vi "Maximum Corr coeff.vi"() -> (5 "Plug in titles":string[](array[string]), 7 "Plug in values":string[](array[string]))   [LabVIEW 2021]
uses:
  Controls/Inst_type.ctl
  <vilib>/Analysis/3filter.llb/Filter Passband Type.ctl
  Globals/Meas_global.vi
  <vilib>/Analysis/3filter.llb/Zero Phase Filter (Cascade, DBL).vi
  <vilib>/Analysis/NI_AALBase.lvlib
panel:
  in  "Inst 2":bool
  in  "X Displacement (mm)":dbl
  out "Values":string[](array[string])
  out "Ch Names":string[](array[string])
  in  "Device ID Contains":string="B2"
  in  "Inject Sync Delay Values":bool
  in  "Minimum Correlation Coefficient\nto give time lag for":dbl=0.1
  in  "Time Trace":bool
  in  "Wind turbine location\n(Applicable only if \nInput own variables? is OFF)":dbl=10000.0
  out "Error":i32
  in  "Filter 2nd Instrument data?":bool
  in  "Freq Cutoff Inst 2":dbl=100.0
  in  "Freq Cutoff Inst 1":dbl=100.0
  in  "Filter 1st Instrument Data?":bool
  in  "Start point(s)":dbl=-1.5
  in  "Time step (s)":dbl=0.05
  in  "Input own variables?":bool=TRUE
  out "Start point":dbl
  out "XY Graph 2":cluster{dbl[], dbl[]}(graph)
  out "Time step":dbl
  in  "Number of estimates":i32=60
  out "Time Trace":cluster{"Time (ms)":dbl[], "Eng Values":dbl[]}[](graph)
  in  "Instrumnt 2":i32=1
  in  "Instrument 1":i32
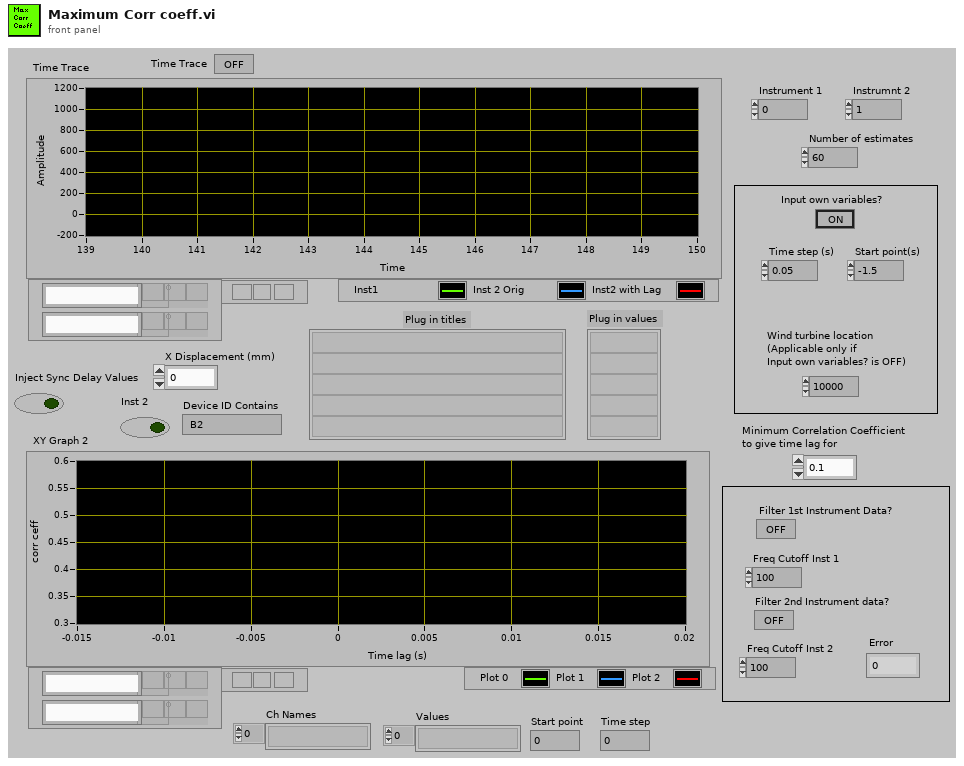
[diagram p1: front panel]
types:
  T1 = typedef "Analysis_info_cluster.ctl" = cluster{"Colour":u32, "Inst type":T2, "Inst name":string, "Symbol":string, "Code name":string, "Extra Info":string, "Inst Array":T3, "Extra Titles":string[], "Extra Values":string[], "U":dbl, "u^2":dbl, "u^3":dbl, "u^4":dbl, "Skew_u":dbl, "Kurt_u":dbl, "Sd Error in Mean":dbl, "% u'/U":dbl, "X":dbl, "Y":dbl, "Z":dbl, "Timescale integral Estimate":dbl, "Sd Error in Variance":dbl, "Calib File":path, "Calib Constants":dbl[], "Output Position":bool, "Stats":enum16{"None", "Basic", "Full"}, "Av Sampling Rate":dbl, "Av No of Samples":dbl, "Total Meas Time (s)":dbl, "ADAM Ch Name":string, "Max value":dbl, "Min value":dbl, "Req Sample Rate Hz":dbl, "Sync Delay Time (s)":dbl, "Ch No":i16, "Device":string, "Use Latest Calib":bool, "Port":string, "Metadata Ch Names":string[], "Metadata Ch Values":string[], "Label":string}
  T2 = typedef "Inst_type.ctl" = enum16{"Raw voltage", "Raw with zero offsetting", "Propeller anemometer", "Pressure Transducer", "Pitot-static tube", "Hot wire", "Cross wire 1", "Cross wire 2", "Generic Linear", "Generic Polynomial", "Generic BackPoly", "Fast FID", "Thermocouple", "Cold wire", "Pulsed Wire", "LDA Vel", "LDA Tran time", "LDA Arr time", "Microphone"}
  T3 = typedef "Instrument_Array.ctl" = enum16{"PWA", "LDA", "Analogue"}
  T4 = typedef "Time_Trace_Cluster.ctl" = cluster{"Weighting":dbl[], "Voltage":dbl[], "Eng Values":dbl[]}
  T5 = enum16{"Save no data", "Save data in new files", "Save data in existing files"}
  T6 = typedef "NI_AALBase.lvlib/Filter Passband Type.ctl" = enum32{"Lowpass", "Highpass", "Bandpass", "Bandstop"}
  T7 = cluster{"sorted array":dbl[], "Eng Values":dbl[]}
  T8 = cluster{"filter structure":enum32{"IIR 2nd Order", "IIR 4th Order"}, "Reverse Coefficients":dbl[], "Forward Coefficients":dbl[]}
  T9 = typedef "Cross_Moments_Shift_Cluster.ctl" = cluster{"Stats":dbl[], "Resampled No of Samples":i32, "Resampled delta T":dbl, "Cross Correlation":dbl[]}
  T10 = typedef "Shift_Cluster.ctl" = cluster{"Stats":dbl[], "Spectra_Auto":dbl[], "Histogram":dbl[], "Hist Max":dbl, "Hist Min":dbl, "No of Samples":i32, "No in plume":i32, "Weight sum":dbl, "No Of Hist bins":i32, "TimeTrace Max":dbl, "Time Trace Min":dbl, "Trace St Deviation":dbl}
  T11 = typedef "Correlation_cluster1.ctl" = cluster{"U inst":string, "uw":dbl, "u^2w":dbl, "uw^2":dbl, "uw/u'w'":dbl, "W inst":string, "uw^3":dbl, "u^3w":dbl, "u^2w^2":dbl, "Index U":i32, "Index W":i32, "Error info":string[], "Paired Sampling Rate (Hz)":dbl, "u^2 Paired":dbl, "w^2 Paired":dbl, "Time Window (ms)":dbl}
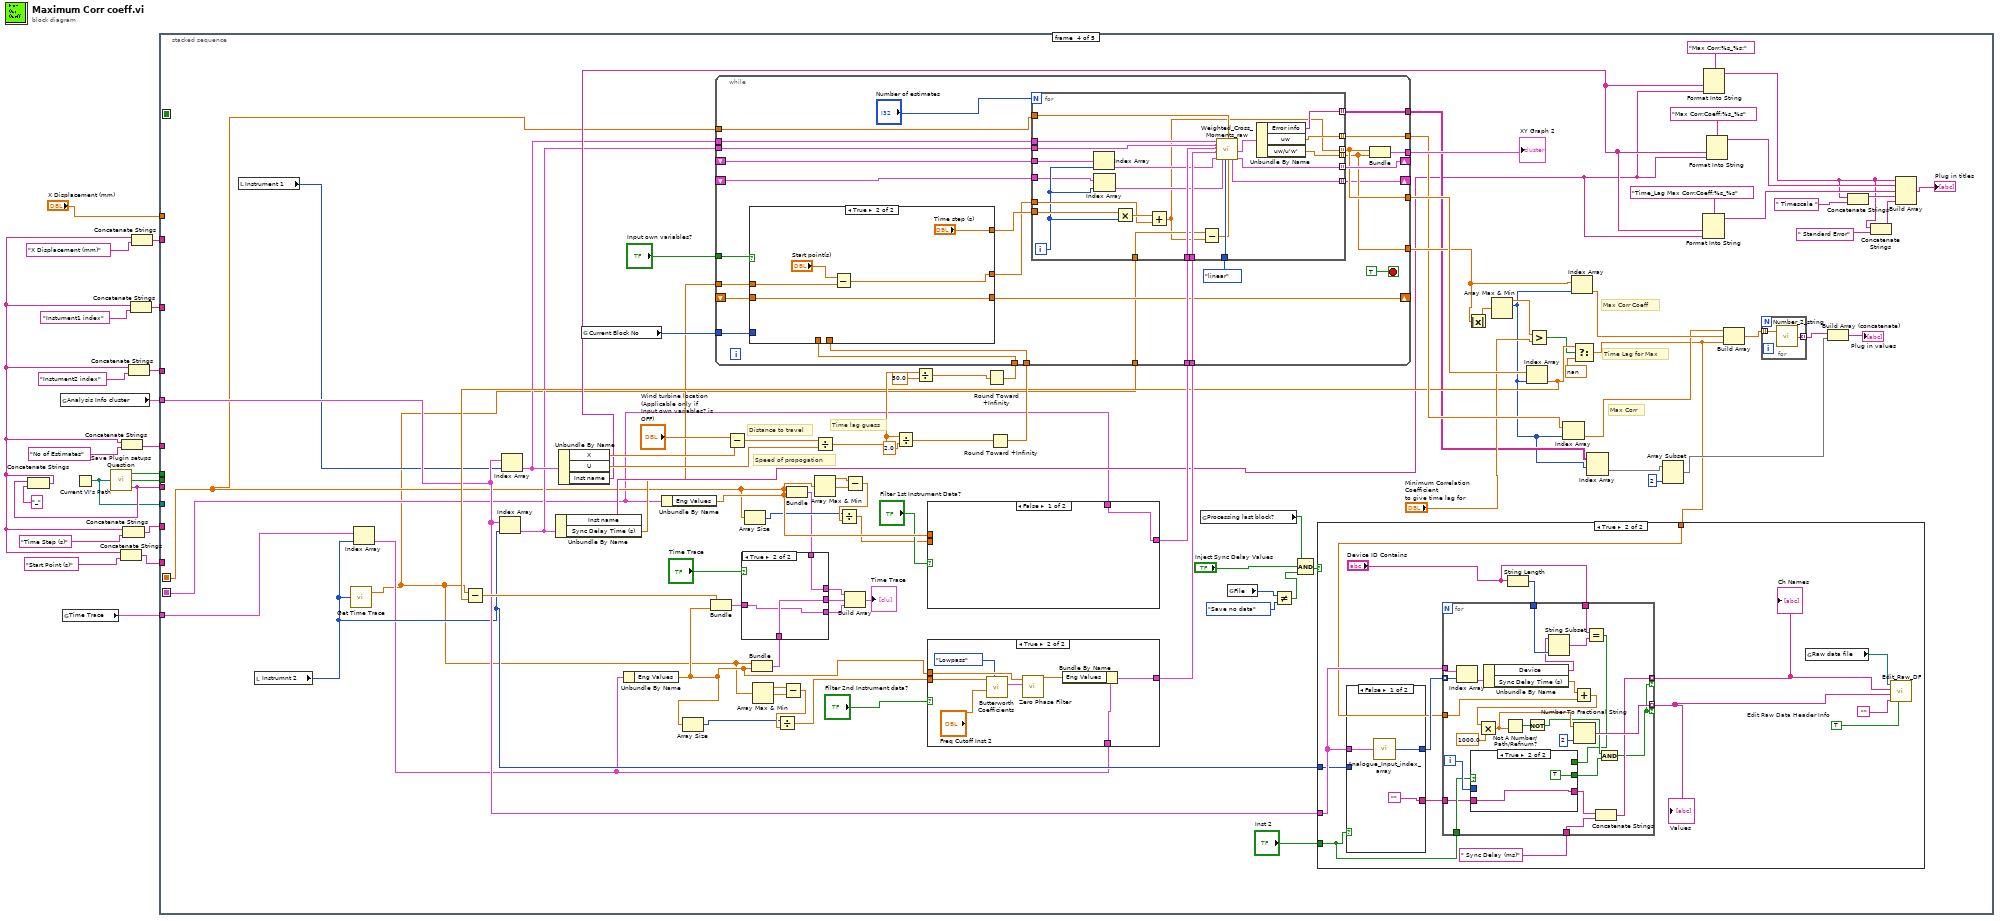
[diagram p0: block diagram]
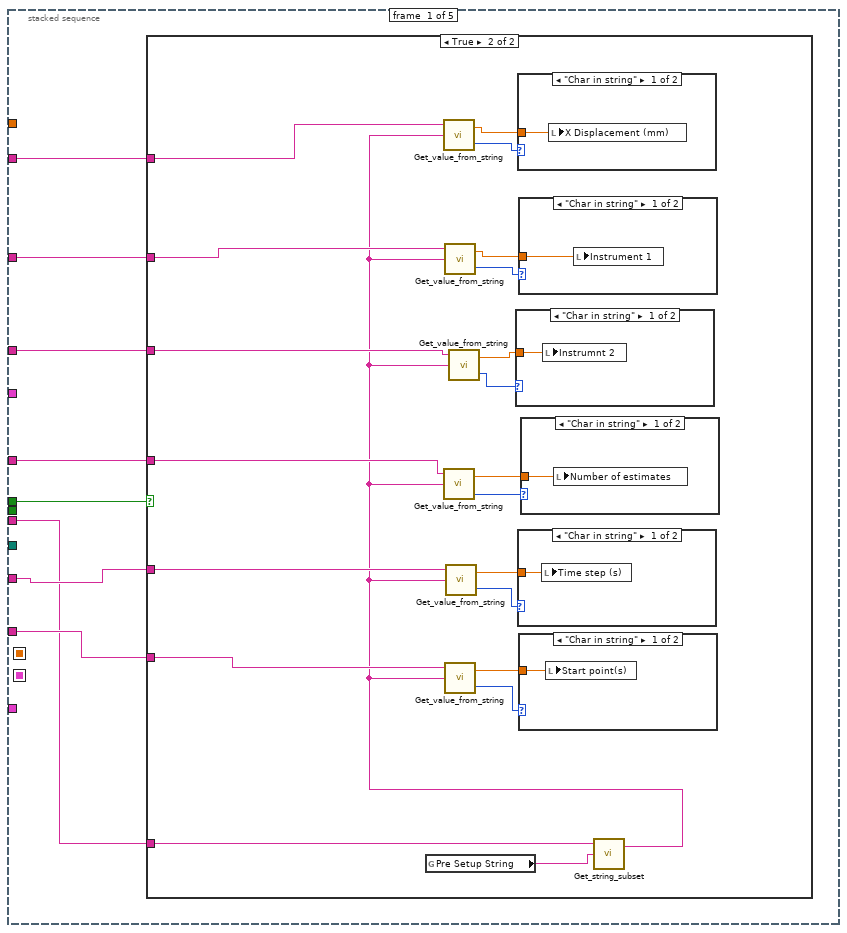
[diagram p2: hidden frame]
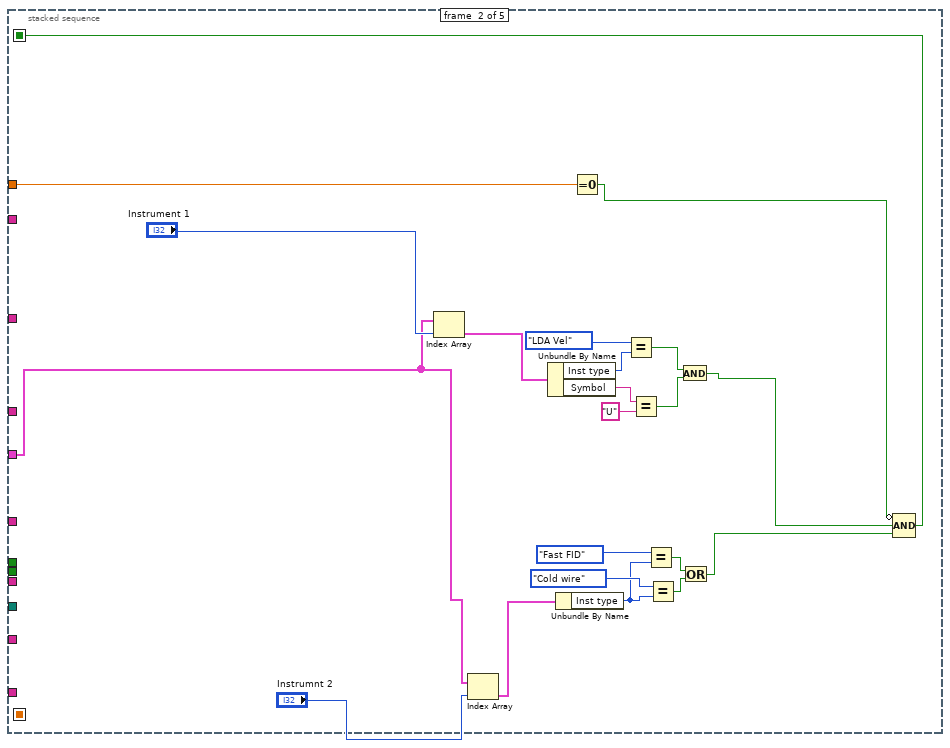
[diagram p10: hidden frame]
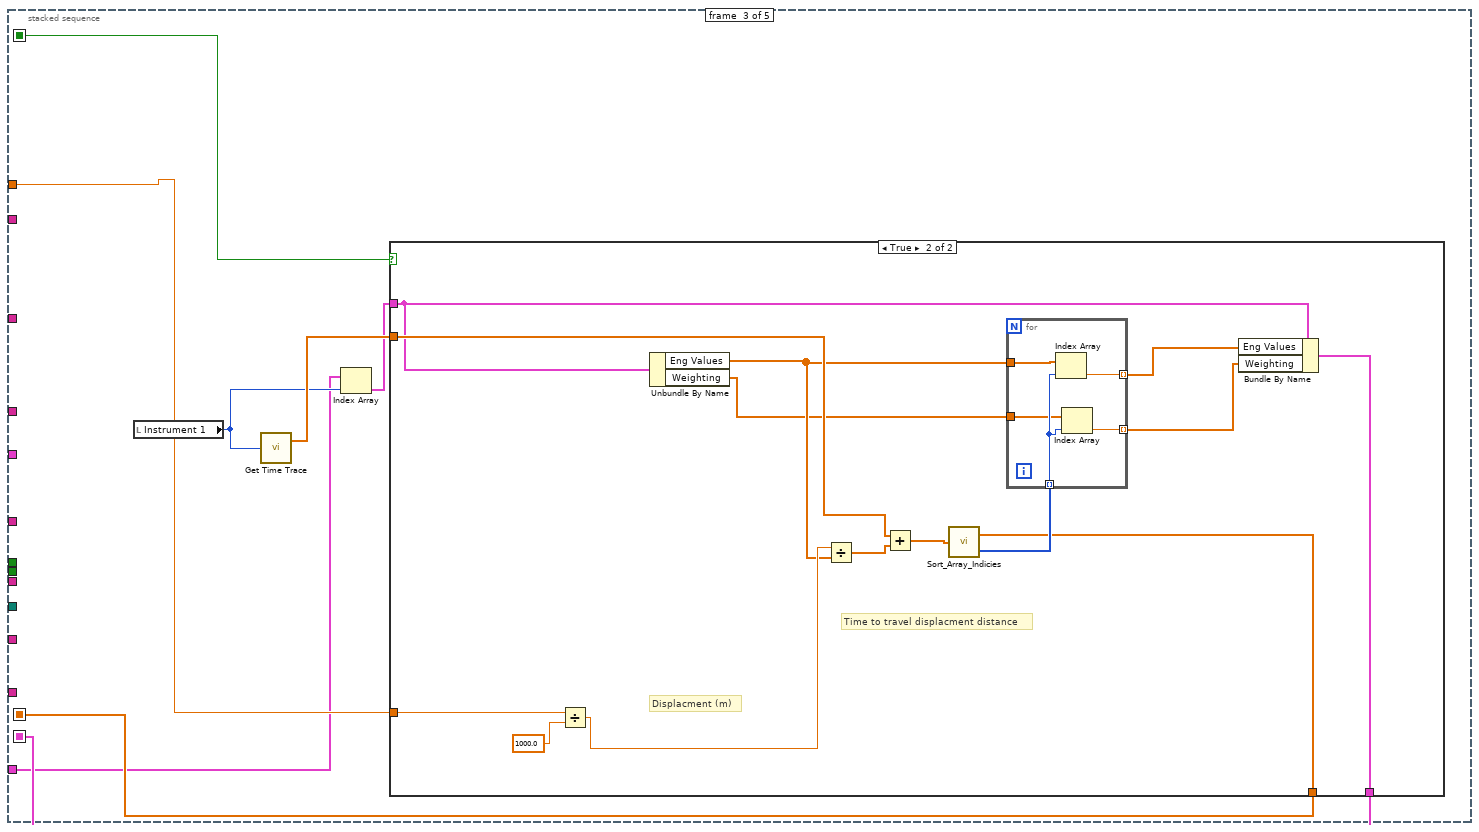
[diagram p11: hidden frame]
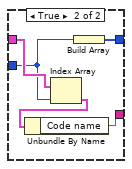
[diagram p14: hidden frame]
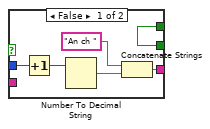
[diagram p15: hidden frame]
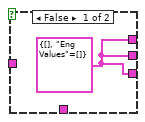
[diagram p16: hidden frame]
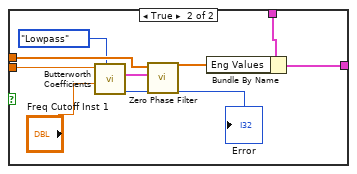
[diagram p18: hidden frame]
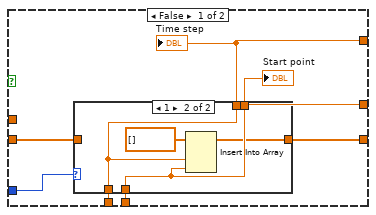
[diagram p19: hidden frame]
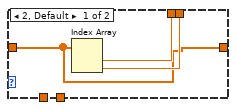
[diagram p20: hidden frame]
diagram:
  n1 = global read "Meas_global.vi" "Analysis Info cluster"() -> (w21:T1[])
  n2 = global read "Meas_global.vi" "Time Trace"() -> (w4:T4[])
  n3 = Current VI's Path() -> (path=w5:path)
  n4 = call "Save Plugin setups Question.vi"("VI path"=w5) -> ("Load Plugin Setup"=w8:bool, "Save Plugin Setup"=w7:bool, "Plugin_Label"=w6:string)
  n5 = Concatenate Strings(w6, "_" ("string")) -> (w2:string)
  n6 = Concatenate Strings(w2, "Start Point (s)" ("Label for value")) -> (w18:string)
  n7 = Concatenate Strings(w2, "No of Estimates" ("Label for value")) -> (w11:string)
  n8 = Concatenate Strings(w2, "Time Step (s)" ("Label for value")) -> (w17:string)
  n9 = Concatenate Strings(w2, "Instument2 index" ("Label for value")) -> (w16:string)
  n10 = Concatenate Strings(w2, "Instument1 index" ("Label for value")) -> (w15:string)
  n11 = Concatenate Strings(w2, "X Displacement (mm)" ("Label for value")) -> (w1:string)
  n12 = stacked-sequence {
    seq-local: [_ w74 _ _ _] -> [_ _ w84 _ _]
    seq-local: [_ _ w82 _ _] -> [_ _ _ w111 _]
    seq-local: [_ _ w80 _ _] -> [_ _ _ w108 _]
    tunnel: w11 -> [w29 _ _ _ w354]
    tunnel: w18 -> [w27 _ _ _ w353]
    tunnel: w17 -> [w28 _ _ _ w352]
    tunnel: w16 -> [w26 _ _ _ w350]
    tunnel: w15 -> [w25 _ _ _ w351]
    tunnel: w21 -> [_ w64 _ w115 _]
    tunnel: "X Displacement (mm)" -> [_ w73 w85 _ _]
    tunnel: w8 -> [w24 _ _ _ _]
    tunnel: w7 -> [_ _ _ _ w349]
    tunnel: w6 -> [w23 _ _ _ w348]
    tunnel: w5 -> [_ _ _ _ w347]
    tunnel: w4 -> [_ _ w79 w112 _]
    tunnel: w1 -> [w22 _ _ _ w346]
    frame #0 {
      n13 = case shown="True" w24 {
        tunnel: w29 -> [_ w49]
        tunnel: w28 -> [_ w48]
        tunnel: w27 -> [_ w47]
        tunnel: w26 -> [_ w38]
        tunnel: w25 -> [_ w37]
        tunnel: w23 -> [_ w34]
        tunnel: w22 -> [_ w31]
        frame False {
        }
        frame True {
          n14 = global read "Meas_global.vi" "Pre Setup String"() -> (w50:string)
          n15 = call "Get_string_subset.vi"("String to split"=w50, "File Label"=w34) -> ("Output string"=w30:string)  [unwired: 2 in, 1 out]
          n16 = call "Get_value_from_string.vi"("Input string"=w30, "Variable name"=w31) -> ("Status"=w32:enum16{"Char in string", "Char not in string"}, "Value"=w33:dbl)  [unwired: 1 in]
          n17 = call "Get_value_from_string.vi"("Input string"=w30, "Variable name"=w49) -> ("Status"=w45:enum16{"Char in string", "Char not in string"}, "Value"=w46:dbl)  [unwired: 1 in]
          n18 = call "Get_value_from_string.vi"("Input string"=w30, "Variable name"=w37) -> ("Status"=w39:enum16{"Char in string", "Char not in string"}, "Value"=w36:dbl)  [unwired: 1 in]
          n19 = call "Get_value_from_string.vi"("Input string"=w30, "Variable name"=w47) -> ("Status"=w42:enum16{"Char in string", "Char not in string"}, "Value"=w43:dbl)  [unwired: 1 in]
          n20 = call "Get_value_from_string.vi"("Input string"=w30, "Variable name"=w48) -> ("Status"=w41:enum16{"Char in string", "Char not in string"}, "Value"=w44:dbl)  [unwired: 1 in]
          n21 = call "Get_value_from_string.vi"("Input string"=w30, "Variable name"=w38) -> ("Status"=w40:enum16{"Char in string", "Char not in string"}, "Value"=w35:dbl)  [unwired: 1 in]
          n22 = case shown="\"Char in string\"" w40 {
            tunnel: w35 -> [w52 _]
            frame "Char in string" {
              n23 = local write "Instrumnt 2"(w52) -> ()
            }
            frame "Char not in string" {
            }
          }
          n24 = case shown="\"Char in string\"" w32 {
            tunnel: w33 -> [w51 _]
            frame "Char in string" {
              n25 = local write "X Displacement (mm)"(w51) -> ()
            }
            frame "Char not in string" {
            }
          }
          n26 = case shown="\"Char in string\"" w41 {
            tunnel: w44 -> [w55 _]
            frame "Char in string" {
              n27 = local write "Time step (s)"(w55) -> ()
            }
            frame "Char not in string" {
            }
          }
          n28 = case shown="\"Char in string\"" w39 {
            tunnel: w36 -> [w53 _]
            frame "Char in string" {
              n29 = local write "Instrument 1"(w53) -> ()
            }
            frame "Char not in string" {
            }
          }
          n30 = case shown="\"Char in string\"" w42 {
            tunnel: w43 -> [w54 _]
            frame "Char in string" {
              n31 = local write "Start point(s)"(w54) -> ()
            }
            frame "Char not in string" {
            }
          }
          n32 = case shown="\"Char in string\"" w45 {
            tunnel: w46 -> [w56 _]
            frame "Char in string" {
              n33 = local write "Number of estimates"(w56) -> ()
            }
            frame "Char not in string" {
            }
          }
        }
      }
    }
    frame #1 {
      n34 = Index Array(array=w64, index="Instrument 1") -> (element=w65:T1)
      n35 = Index Array(array=w64, index="Instrumnt 2") -> (element=w57:T1)
      n36 = Unbundle By Name(w65) -> ("Inst type"=w70:T2, "Symbol"=w69:string)
      n37 = Unbundle By Name(w57) -> ("Inst type"=w60:T2)
      n38 = Equal To 0?(x=w73) -> (x = 0?=w75:bool)
      n39 = Equal?(x=Inst_type."LDA Vel" ("Inst type"), y=w70) -> (x = y?=w66:bool)
      n40 = Equal?(x=w69, y="U") -> (x = y?=w67:bool)
      n41 = Equal?(x=Inst_type."Fast FID" ("Inst type"), y=w60) -> (x = y?=w59:bool)
      n42 = Equal?(x=Inst_type."Cold wire" ("Inst type"), y=w60) -> (x = y?=w58:bool)
      n43 = And(x=w66, y=w67) -> (x .and. y?=w76:bool)
      n44 = Or(x=w59, y=w58) -> (x .or. y?=w77:bool)
      n45 = Compound Arithmetic op=AND(invert w75, w76, w77) -> (w74:bool)
    }
    frame #2 {
      n46 = local read "Instrument 1"() -> (w81:i32)
      n47 = call "Get Time Trace.vi"("Channel Index"=w81) -> ("Time (s)"=w83:dbl[])  [unwired: 1 out]
      n48 = Index Array(array=w79, index=w81) -> (element=w78:T4)
      n49 = case shown="True" w84 {
        tunnel: w85 -> [_ w99]
        tunnel: w83 -> [w87 w97]
        tunnel: [w87 w89] -> w82
        tunnel: [w86 w90] -> w80
        tunnel: w78 -> [w86 w88]
        frame False {
        }
        frame True {
          # "Displacment (m)"
          # "Time to travel displacment distance"
          n50 = Divide(x=w99, y=1000.0) -> (x/y=w100:dbl)
          n51 = Unbundle By Name(w88) -> ("Eng Values"=w94:dbl[], "Weighting"=w92:dbl[])
          n52 = Divide(x=w100, y=w94) -> (x/y=w98:dbl[])
          n53 = Add(x=w97, y=w98) -> (x+y=w96:dbl[])
          n54 = call "Sort_Array_Indicies.vi"("unsorted array"=w96) -> ("sorted array"=w89:dbl[], "Sort Index"=w95:i32[])
          n55 = for {
            tunnel: w95 -> [w104] mode=indexing
            tunnel: w94 -> [w106]
            tunnel: [w105] -> w93 mode=indexing
            tunnel: w92 -> [w103]
            tunnel: [w102] -> w91 mode=indexing
            n56 = Index Array(array=w106, index=w104) -> (element=w105:dbl)
            n57 = Index Array(array=w103, index=w104) -> (element=w102:dbl)
          }
          n58 = Bundle By Name(cluster=w88, "Eng Values"=w93, "Weighting"=w91) -> (w90:T4)
        }
      }
    }
    frame #3 {
      # "Max Corr"
      # "Time Lag for Max"
      # "Max Corr Coeff"
      # "Speed of propogation"
      # "Distance to travel"
      # "Time lag guess"
      n59 = local read "Instrument 1"() -> (w113:i32)
      n60 = local read "Instrumnt 2"() -> (w110:i32)
      n61 = call "Get Time Trace.vi"("Channel Index"=w110) -> ("Time (s)"=w107:dbl[])  [unwired: 1 out]
      n62 = Index Array(array=w112, index=w110) -> (element=w109:T4)
      n63 = Index Array(array=w115, index=w110) -> (element=w137:T1)
      n64 = Index Array(array=w115, index=w113) -> (element=w138:T1)
      n65 = Unbundle By Name(w137) -> ("Inst name"=w124:string, "Sync Delay Time (s)"=w116:dbl)
      n66 = Unbundle By Name(w138) -> ("X"=w169:dbl, "U"=w168:dbl, "Inst name"=w145:string)
      n67 = global read "Meas_global.vi" "Current Block No"() -> (w191:i32)
      n68 = Unbundle By Name(w109) -> ("Eng Values"=w183:dbl[])
      n69 = Unbundle By Name(w108) -> ("Eng Values"=w188:dbl[])
      n70 = Array Size(array=w183) -> (size(s)=w171:i32)
      n71 = Subtract(x="Wind turbine location\n(Applicable only if \nInput own variables? is OFF)", y=w169) -> (x-y=w167:dbl)
      n72 = Array Size(array=w111) -> (size(s)=w177:i32)
      n73 = Bundle("Time (s)"=w107, "Eng Values"=w183) -> (w150:cluster{"Time (s)":dbl[], "Eng Values":dbl[]})  [unwired: 1 in]
      n74 = Array Max & Min(array=w107) -> (max value=w173:dbl, min value=w174:dbl)  [unwired: 2 out]
      n75 = Subtract(x=w173, y=w174) -> (x-y=w172:dbl)
      n76 = Divide(x=w171, y=w172) -> (x/y=w175:dbl)
      n77 = Bundle("sorted array"=w111, "Eng Values"=w188) -> (w153:T7)  [unwired: 1 in]
      n78 = Divide(x=w167, y=w168) -> (x/y=w193:dbl)
      n79 = Array Max & Min(array=w111) -> (max value=w180:dbl, min value=w179:dbl)  [unwired: 2 out]
      n80 = Subtract(x=w180, y=w179) -> (x-y=w178:dbl)
      n81 = Divide(x=w177, y=w178) -> (x/y=w176:dbl)
      n82 = Divide(x=w193, y=2.0) -> (x/y=w165:dbl)
      n83 = Divide(x=w193, y=50.0) -> (x/y=w164:dbl)
      n84 = case shown="False" "Filter 1st Instrument Data?" {
        tunnel: w188 -> [_ w275]
        tunnel: w176 -> [_ w274]
        tunnel: w108 -> [w267 w272]
        tunnel: [w267 w271] -> w187
        frame False {
        }
        frame True {
          n85 = call <vilib>:"Butterworth Coefficients.vi"("filter type"=Filter_Passband_Type."Lowpass", "low cutoff freq: fl"="Freq Cutoff Inst 1", "sampling freq: fs"=w274) -> ("error"=→"Error":i32, "IIR Filter Cluster"=w276:T8)  [unwired: 7 in]
          n86 = call-poly <vilib>:"Zero Phase Filter.vi"("IIR Filter Cluster"=w276, "X"=w275) -> ("Filtered X"=w273:dbl[])  [unwired: 8 in, 1 out]
          n87 = Bundle By Name(cluster=w272, "Eng Values"=w273) -> (w271:T4)
        }
      }
      n88 = case shown="True" "Filter 2nd Instrument data?" {
        tunnel: w183 -> [_ w265]
        tunnel: w175 -> [_ w264]
        tunnel: [w258 w262] -> w182
        tunnel: w109 -> [w258 w260]
        frame False {
        }
        frame True {
          n89 = call <vilib>:"Butterworth Coefficients.vi"("filter type"=Filter_Passband_Type."Lowpass", "low cutoff freq: fl"="Freq Cutoff Inst 2", "sampling freq: fs"=w264) -> ("IIR Filter Cluster"=w266:T8)  [unwired: 7 in, 1 out]
          n90 = call-poly <vilib>:"Zero Phase Filter.vi"("IIR Filter Cluster"=w266, "X"=w265) -> ("Filtered X"=w263:dbl[])  [unwired: 8 in, 1 out]
          n91 = Bundle By Name(cluster=w260, "Eng Values"=w263) -> (w262:T4)
        }
      }
      n92 = Round Toward +Infinity(x=w164) -> (ceil(x): smallest int >= x=w163:dbl)
      n93 = Round Toward +Infinity(x=w165) -> (ceil(x): smallest int >= x=w166:dbl)
      n94 = while {
        tunnel: w187 -> [w303]
        tunnel: w182 -> [w302]
        shift-right: [w300] -> _
        shift-left: _ -> [w299]
        tunnel: [w298] -> w195
        tunnel: [w296] -> w189
        tunnel: [w289] -> w181
        tunnel: w163 -> [w294]
        tunnel: w191 -> [w295]
        tunnel: w166 -> [w293]
        shift-right: [w292] -> _
        shift-left: _ -> [w291]
        tunnel: "Input own variables?" -> [w288]
        tunnel: [w286] -> w147
        tunnel: w138 -> [w285]
        tunnel: w137 -> [w284]
        tunnel: [w283] -> w136
        tunnel: w116 -> [w282]
        shift-right: [w280] -> _
        shift-left: _ -> [w279]
        tunnel: w111 -> [w278]
        tunnel: w107 -> [w277]
        stop <- TRUE stop-if-true
        n95 = case shown="True" w288 {
          tunnel: w295 -> [w310 _]
          tunnel: w294 -> [w309 _]
          tunnel: w293 -> [w308 _]
          tunnel: [w307 w321] -> w292
          tunnel: w291 -> [w306 w321]
          tunnel: [w305 w318] -> w287
          tunnel: [w304 "Time step (s)"] -> w290
          tunnel: w282 -> [_ w319]
          frame False {
            n96 = case shown="1" w310 {
              tunnel: w309 -> [_ w316]
              tunnel: [w313 w316] -> w304
              tunnel: [w312 w317] -> w305
              tunnel: w308 -> [_ w317]
              tunnel: [w311 w315] -> w307
              tunnel: w306 -> [w311 _]
              frame 2, Default {
                n97 = Index Array(array=w311) -> (element #1=w313:dbl, element #2=w312:dbl)  [unwired: 2 in]
              }
              frame 1 {
                n98 = Insert Into Array(array=dbl[] [], new element #1=w316, new element #2=w317) -> (w315:dbl[])  [unwired: 1 in]
              }
            }
            "Time step" <- w304
            "Start point" <- w305
          }
          frame True {
            n99 = Subtract(x="Start point(s)", y=w319) -> (x-y=w318:dbl)
          }
        }
        n100 = for {
          N: "Number of estimates" -> [_]
          tunnel: w303 -> [w336]
          tunnel: w302 -> [w335]
          tunnel: w290 -> [w345]
          tunnel: [w333] -> w300 mode=indexing
          tunnel: w299 -> [w344]
          tunnel: [w324] -> w296 mode=indexing
          tunnel: [w343] -> w289 mode=indexing
          tunnel: w287 -> [w341]
          tunnel: [w340] -> w286 mode=indexing
          tunnel: w285 -> [w338]
          tunnel: w284 -> [w337]
          tunnel: [w339] -> w283 mode=indexing
          tunnel: enum16{"nearest", "linear"}."linear" ("interp. method") -> [w326]
          tunnel: [w331] -> w280 mode=indexing
          tunnel: w279 -> [w329]
          tunnel: w278 -> [w327]
          tunnel: w277 -> [w325]
          i -> [w330]
          n101 = Index Array(array=w344, index=w330) -> (element=w332:T9)
          n102 = Index Array(array=w329, index=w330) -> (element=w328:T10)
          n103 = Multiply(x=w345, y=w330) -> (x*y=w342:dbl)
          n104 = Add(x=w342, y=w341) -> (x+y=w324:dbl)
          n105 = Subtract(x=w325, y=w324) -> (x-y=w323:dbl[])
          n106 = call "Weighted_Cross_Moments_raw.vi"("AI Cluster 1"=w338, "AI Cluster 2"=w337, "Time Cluster 1"=w336, "Time Cluster 2"=w335, "Shift Cluster In"=w332, "Shift Input"=w328, "interp. method"=w326, "Time (s) 1"=w327, "Time (s) 2"=w323) -> ("Shift Output"=w331:T10, "output cluster"=w334:T11, "Shift Cluster Out"=w333:T9)  [unwired: 8 in]
          n107 = Unbundle By Name(w334) -> ("Error info"=w339:string[], "uw"=w340:dbl, "uw/u'w'"=w343:dbl)
        }
        n108 = Bundle(w296, w289) -> (w298:cluster{dbl[], dbl[]})  [unwired: 1 in]
      }
      "XY Graph 2" <- w195
      n109 = global read "Meas_global.vi" "Processing last block?"() -> (w117:bool)
      n110 = global read "Meas_global.vi" "File"() -> (w121:T5)
      n111 = Not Equal?(x=w121, y=T5."Save no data" ("File")) -> (x != y?=w120:bool)
      n112 = Compound Arithmetic op=AND(w117, "Inject Sync Delay Values", w120) -> (w118:bool)
      n113 = Absolute Value(x=w181) -> (abs(x)=w184:dbl[])
      n114 = Array Max & Min(array=w184) -> (max value=w143:dbl, max index (indices)=w135:i32)  [unwired: 2 out]
      n115 = Index Array(array=w189, index=w135) -> (element=w141:dbl)
      n116 = Subtract(x=w107, y=w141) -> (x-y=w155:dbl[])
      n117 = Bundle(w155, "Eng Values"=w183) -> (w149:cluster{dbl[], "Eng Values":dbl[]})  [unwired: 1 in]
      n118 = case shown="True" "Time Trace" {
        tunnel: w153 -> [_ w255]
        tunnel: [w252 w255] -> w152
        tunnel: [w252 w254] -> w151
        tunnel: w150 -> [_ w254]
        tunnel: w149 -> [_ w253]
        tunnel: [w252 w253] -> w148
        frame False {
          w252 = cluster{dbl[], "Eng Values":dbl[]} {[], "Eng Values"=[]}
        }
        frame True {
        }
      }
      n119 = Build Array(w152, w151, w148) -> (→"Time Trace":cluster{"Time (s)":dbl[], "Eng Values":dbl[]}[])
      n120 = Greater?(x=w143, y="Minimum Correlation Coefficient\nto give time lag for") -> (0:w140:bool)
      n121 = Index Array(array=w147, index=w135) -> (element=w144:dbl)
      n122 = Index Array(array=w181, index=w135) -> (element=w161:dbl)
      n123 = Select(t=w141, s=w140, f=nan) -> (s? t:f=w123:dbl)
      n124 = case shown="True" w118 {
        tunnel: w115 -> [_ w208]
        tunnel: w123 -> [_ w205]
        tunnel: "Inst 2" -> [_ w200]
        tunnel: w110 -> [_ w202]
        frame False {
        }
        frame True {
          w203 = TRUE  # Edit Raw Data Header Info
          n125 = case shown="False" w200 {
            tunnel: w208 -> [w213 w217]
            tunnel: [w212 w218] -> w207
            tunnel: w202 -> [_ w216]
            tunnel: ["" w214] -> w198
            frame False {
              n126 = call "Analogue_Input_index_array.vi"("Analysis Info cluster"=w213) -> ("Array"=w212:i32[])
            }
            frame True {
              n127 = Index Array(array=w217, index=w216) -> (element=w215:T1)
              n128 = Unbundle By Name(w215) -> ("Code name"=w214:string)
              n129 = Build Array(w216) -> (w218:i32[])
            }
          }
          n130 = String Length(string="Device ID Contains") -> (length=w210:i32)
          n131 = for {
            tunnel: w208 -> [w240]
            tunnel: w210 -> [w243]
            tunnel: "Device ID Contains" -> [w241]
            tunnel: w207 -> [w239] mode=indexing
            tunnel: [w224] -> w199 mode=indexing if=w221
            tunnel: [w228] -> w206 mode=indexing if=w221
            tunnel: w205 -> [w234]
            tunnel: " Sync Delay (ms)" -> [w226]
            tunnel: w200 -> [w227]
            tunnel: w198 -> [w223]
            i -> [w237]
            n132 = Index Array(array=w240, index=w239) -> (element=w238:T1)
            n133 = Unbundle By Name(w238) -> ("Device"=w236:string, "Sync Delay Time (s)"=w235:dbl)
            n134 = String Subset(string=w236, length (rest)=w243) -> (substring=w242:string)  [unwired: 1 in]
            n135 = Add(x=w235, y=w234) -> (x+y=w230:dbl)
            n136 = Multiply(x=w230, y=1000.0) -> (x*y=w229:dbl)
            n137 = Not A Number/Path/Refnum?(number/path/refnum=w229) -> (NaN/Path/Refnum?=w233:bool)
            n138 = Not(x=w233) -> (.not. x?=w220:bool)
            n139 = Number To Fractional String(number=w229, precision (6)=i16 2) -> (F-format string=w228:string)  [unwired: 2 in]
            n140 = Equal?(x=w241, y=w242) -> (x = y?=w219:bool)
            n141 = case shown="True" w227 {
              tunnel: w237 -> [w246 _]
              tunnel: [w245 w251] -> w225
              tunnel: w223 -> [_ w251]
              tunnel: [w244 TRUE] -> w222
              tunnel: w219 -> [w244 _]
              frame False {
                n142 = Increment(x=w246) -> (x+1=w249:i32)
                n143 = Number To Decimal String(number=w249) -> (decimal integer string=w248:string)  [unwired: 1 out]
                n144 = Concatenate Strings("An ch ", w248) -> (w245:string)
              }
              frame True {
              }
            }
            n145 = Concatenate Strings(w225, w226) -> (w224:string)
            n146 = And(x=w220, y=w222) -> (x .and. y?=w221:bool)
          }
          "Ch Names" <- w199
          "Values" <- w206
          n147 = global read "Meas_global.vi" "Raw data file"() -> (w204:path)
          n148 = call "Edit_Raw_DF.vi"("Edit Raw Data Header Info"=w203, "New Analysis Info Cluster Setup"="", "New Values In"=w206, "New Chs In"=w199, "Data filename"=w204) -> ()  [unwired: 1 in, 4 out]
        }
      }
      n149 = Index Array(array=w136, index (row)=w135) -> (element=w130:string[])  [unwired: 1 in]
      n150 = Array Subset(array=w130, length=2) -> (w128:string[])  [unwired: 1 in]
      n151 = Format Into String(format string="Time_Lag Max Corr:Coeff:%s_%s", w145, w124) -> (resulting string=w156:string)  [unwired: 2 in, 1 out]
      n152 = Format Into String(format string="Max Corr:%s_%s:", w145, w124) -> (resulting string=w126:string)  [unwired: 2 in, 1 out]
      n153 = Format Into String(format string="Max Corr:Coeff:%s_%s", w145, w124) -> (resulting string=w158:string)  [unwired: 2 in, 1 out]
      n154 = Build Array(w144, w161, w123) -> (w162:dbl[])
      n155 = for {
        tunnel: w162 -> [w256] mode=indexing
        tunnel: [w257] -> w134 mode=indexing
        n156 = call "Number_2_string.vi"("number"=w256) -> ("String"=w257:string)  [unwired: 1 in]
      }
      n157 = Build Array (concatenate)(w134, w128) -> (→"Plug in values":string[])
      n158 = Concatenate Strings(w126, " Timescale ") -> (w132:string)
      n159 = Concatenate Strings(w126, " Standard Error") -> (w125:string)
      n160 = Build Array(w126, w158, w156, w132, w125) -> (→"Plug in titles":string[])
    }
    frame #4 {
      n161 = case shown="True" w349 {
        tunnel: w348 -> [_ w359]
        tunnel: w354 -> [_ w374]
        tunnel: w353 -> [_ w371]
        tunnel: w352 -> [_ w370]
        tunnel: w351 -> [_ w364]
        tunnel: w350 -> [_ w363]
        tunnel: w347 -> [_ w358]
        tunnel: w346 -> [_ w356]
        frame False {
        }
        frame True {
          n162 = local read "Number of estimates"() -> (w375:i32)
          n163 = local read "X Displacement (mm)"() -> (w357:dbl)
          n164 = local read "Instrument 1"() -> (w365:i32)
          n165 = local read "Start point(s)"() -> (w373:dbl)
          n166 = local read "Time step (s)"() -> (w372:dbl)
          n167 = local read "Instrumnt 2"() -> (w366:i32)
          n168 = call "Value_to_string.vi"("Value"=w357, "Label for value"=w356) -> ("Output string"=w355:string)  [unwired: 1 in]
          n169 = call "Value_to_string.vi"("Value"=w375, "Label for value"=w374) -> ("Output string"=w369:string)  [unwired: 1 in]
          n170 = call "Value_to_string.vi"("Value"=w365, "Label for value"=w364) -> ("Output string"=w362:string)  [unwired: 1 in]
          n171 = call "Value_to_string.vi"("Value"=w372, "Label for value"=w370) -> ("Output string"=w368:string)  [unwired: 1 in]
          n172 = call "Value_to_string.vi"("Value"=w373, "Label for value"=w371) -> ("Output string"=w367:string)  [unwired: 1 in]
          n173 = call "Value_to_string.vi"("Value"=w366, "Label for value"=w363) -> ("Output string"=w361:string)  [unwired: 1 in]
          n174 = Concatenate Strings(w355, w362, w361, w369, w368, w367) -> (w360:string)
          n175 = call "Save Plugin Setup String.vi"("Plug In Pathname"=w358, "Setup String to Save"=w360, "PlugIn Label"=w359) -> ()  [unwired: 2 in]
        }
      }
    }
  }
